vi "Count Port Lines.vi"(10 "Port":i32, 11 "ActiveDev":tag) -> (3 "# Lines":i32)   [LabVIEW 2020, in "VolatusDAQ.lvlib" / "DAQmxDI.lvclass"]
uses:
  DAQmxDI.lvclass
  DAQmxDI.lvclass/DAQmxDI.ctl
  <resource>/objmgr/daqmx.rc
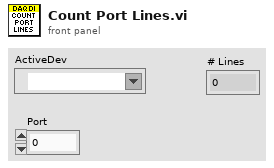
[diagram p1: front panel]
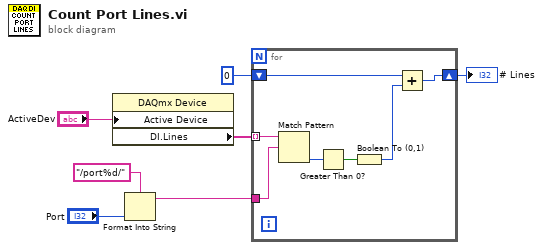
[diagram p0: block diagram]
diagram:
  n1 = property class="DAQmx Device"("Active Device"="ActiveDev") -> ("DI.Lines"=w7:tag[])  [unwired: 2 in, 2 out]
  n2 = Format Into String(format string="/port%d/", "Port") -> (resulting string=w4:string)  [unwired: 2 in, 1 out]
  n3 = for {
    tunnel: w7 -> [w14] mode=indexing
    tunnel: w4 -> [w13]
    shift-right: [w8] -> w2
    shift-left: 0 -> [w10]
    n4 = Match Pattern(string=w14, regular expression=w13) -> (offset past match=w12:i32)  [unwired: 1 in, 3 out]
    n5 = Greater Than 0?(x=w12) -> (x > 0?=w11:bool)
    n6 = Boolean To (0,1)(Boolean=w11) -> (0, 1=w9:i16)
    n7 = Add(x=w10, y=w9) -> (x+y=w8:i32)
  }
  "# Lines" <- w2
